vi "Databasecration.vi"(4 "wait control":u32, 6 "Monedas10":dbl, 7 "Monedas2":dbl, 8 "Monedas1":dbl, 9 "Monedas5":dbl, 10 "NumeroM":i64, 11 "dinero":dbl) -> ()   [LabVIEW 2019]
uses:
  <vilib>/drjdpowell/SQLite Library/SQL Statement/SQL Statement.lvclass/SQL Statement.ctl
  <vilib>/drjdpowell/SQLite Library/SQL Connection/Open (path).vi
  <vilib>/drjdpowell/SQLite Library/SQL Statement/Bind Timestamp (Local Time Offset).vi
  <vilib>/drjdpowell/SQLite Library/SQL Statement/Bind Real.vi
  <vilib>/drjdpowell/SQLite Library/SQL Statement/Bind Integer.vi
  <vilib>/drjdpowell/SQLite Library/SQL Connection/Open (string).vi
  <vilib>/drjdpowell/SQLite Library/SQL Statement/Step.vi
  <vilib>/drjdpowell/SQLite Library/SQL Statement/Bind Text.vi
  <vilib>/JDP Science/JDP Science Common Utilities/Timestamp/Timestamp to Text.vi
  <vilib>/AdvancedString/Path To Command Line String.vi
  <vilib>/drjdpowell/SQLite Library/SQL Statement/Error Message.vi
  <vilib>/drjdpowell/SQLite Library/SQL Connection/Connection.lvclass
  <vilib>/drjdpowell/SQLite Library/SQL Statement/SQL Statement.lvclass
  <vilib>/drjdpowell/SQLite Library/Transaction Helpers/Transaction.lvlib
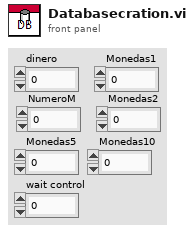
[diagram p1: front panel]
types:
  T1 = enum16{"New or existing", "Existing", "Read only"}
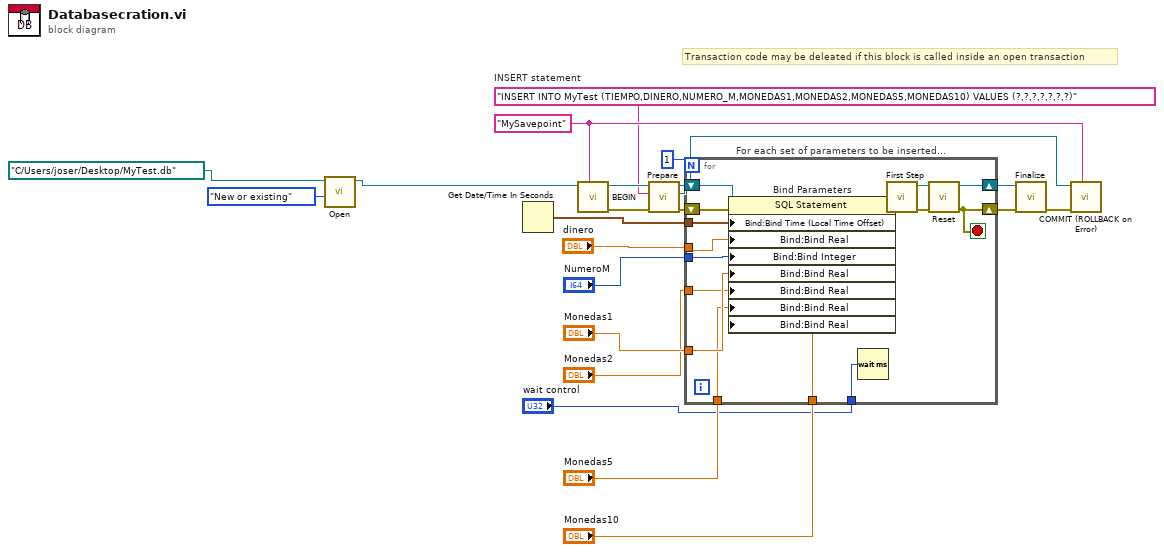
[diagram p0: block diagram]
diagram:
  w19 = "MySavepoint" ("Savepoint name")
  w14 = "INSERT INTO MyTest (TIEMPO,DINERO,NUMERO_M,MONEDAS1,MONEDAS2,MONEDAS5,MONEDAS10) VALUES (?,?,?,?,?,?,?)"  # INSERT statement
  # "Transaction code may be deleated if this block is called inside an open transaction"
  n1 = call-poly <vilib>:"Open.vi"("File Option"=T1."New or existing", "db file"=path "C:/Users/joser/Desktop/MyTest.db") -> ("SQLite Connection"=w22:refnum<class "Connection.lvclass">)  [unwired: 8 in, 1 out]
  n2 = Get Date/Time In Seconds() -> (seconds since 1Jan1904=w8:timestamp)
  n3 = call <vilib>:"BEGIN.vi"("Savepoint name"=w19, "SQLite Connection in"=w22) -> ("error out"=w18:errorcluster, "SQLite Connection"=w17:refnum<class "Connection.lvclass">)  [unwired: 8 in]
  n4 = call <vilib>:"Prepare.vi"("error in (no error)"=w18, "SQL"=w14, "SQLite Connection in"=w17) -> ("error out"=w13:errorcluster, "SQL Statement"=w12:refnum<class "SQL Statement.lvclass">, "SQLite Connection"=w20:refnum<class "Connection.lvclass">)  [unwired: 4 in, 2 out]
  n5 = for "For each set of parameters to be inserted..." {
    N: 1 -> [_]
    shift-right: [w32] -> w15
    shift-left: w12 -> [w38]
    shift-right: [w31] -> w16
    shift-left: w13 -> [w35]
    tunnel: w8 -> [w30]
    tunnel: "dinero" -> [w29]
    tunnel: "NumeroM" -> [w28]
    tunnel: "Monedas1" -> [w27]
    tunnel: "Monedas2" -> [w26]
    tunnel: "Monedas5" -> [w25]
    tunnel: "Monedas10" -> [w24]
    tunnel: "wait control" -> [w23]
    stop <- w31 stop-if-true
    n6 = property on="Bind Parameters" class="SQL Statement"(reference=w38, error in=w35, "Bind:Bind Time (Local Time Offset)"=w30, "Bind:Bind Real"=w29, "Bind:Bind Integer"=w28, "Bind:Bind Real"=w27, "Bind:Bind Real"=w26, "Bind:Bind Real"=w25, "Bind:Bind Real"=w24) -> (reference out=w37:refnum<class "SQL Statement.lvclass">, error out=w36:errorcluster)
    n7 = Wait (ms)(milliseconds to wait=w23) -> ()  [unwired: 1 out]
    n8 = call <vilib>:"First Step.vi"("error in (no error)"=w36, "SQL Statement in"=w37) -> ("error out"=w34:errorcluster, "SQL Statement"=w33:refnum<class "SQL Statement.lvclass">)  [unwired: 7 in, 1 out]
    n9 = call <vilib>:"Reset.vi"("error in (no error)"=w34, "SQL Statement in"=w33) -> ("error out"=w31:errorcluster, "SQL Statement"=w32:refnum<class "SQL Statement.lvclass">)  [unwired: 8 in]
  }
  n10 = call <vilib>:"Finalize.vi"("error in (no error)"=w16, "SQL Statement in"=w15) -> ("error out"=w21:errorcluster)  [unwired: 9 in]
  n11 = call <vilib>:"COMMIT (ROLLBACK on Error).vi"("Savepoint name"=w19, "error in (no error)"=w21, "SQLite Connection in"=w20) -> ()  [unwired: 7 in, 2 out]
